vi "Center Graph.vi"() -> ()   [LabVIEW 2014]
panel:
  in  "# of points":i32
  out "Waveform Graph":dbl[](graph)
  in  "Wave":waveform(dbl)
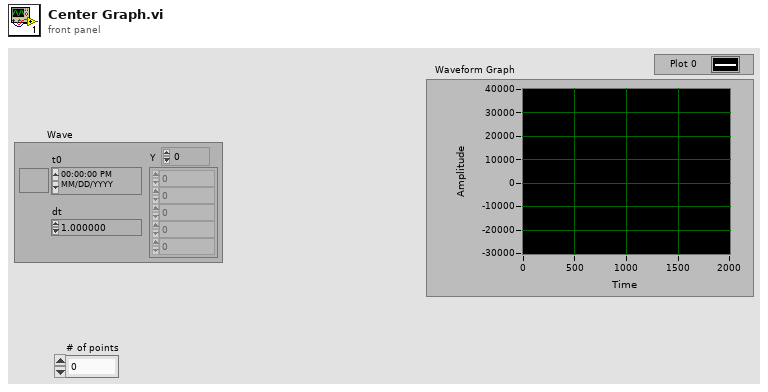
[diagram p1: front panel]
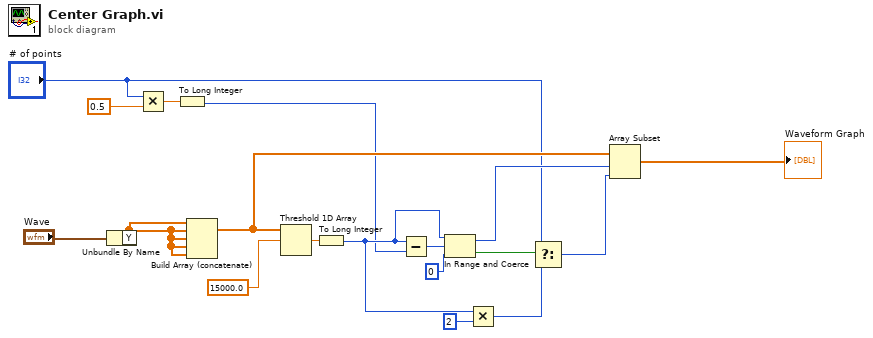
[diagram p0: block diagram]
diagram:
  n1 = Unbundle By Name("Wave") -> ("Y"=w17:dbl[])
  n2 = Multiply(x="# of points", y=0.5) -> (x*y=w2:dbl)
  n3 = To Long Integer(number=w2) -> (32bit integer=w1:i32)
  n4 = Build Array (concatenate)(w17, w17, w17, w17, w17) -> (w8:dbl[])
  n5 = Threshold 1D Array(2:15000.0 ("threshold y"), 3:w8) -> (0:w15:dbl)  [unwired: 1 in]
  n6 = To Long Integer(number=w15) -> (32bit integer=w6:i32)
  n7 = Subtract(x=w6, y=w1) -> (x-y=w10:i32)
  n8 = In Range and Coerce(upper limit=w6, x=w10, lower limit=0) -> (coerced(x)=w13:i32, In Range?=w12:bool)
  n9 = Multiply(x=w6, y=2) -> (x*y=w9:i32)
  n10 = Select(t="# of points", s=w12, f=w9) -> (s? t:f=w11:i32)
  n11 = Array Subset(array=w8, index=w13, length=w11) -> (→"Waveform Graph":dbl[])
